vi "Network-Order Bytes To Words I64.vi"(1 "bytes in":u8[](array[numeric]) format="%02x") -> (0 "words out":i64[](array[numeric]) format="%x")   [LabVIEW 2020, in "NI_Bit Manipulation.lvlib"]
uses:
  <vilib>/Bit Manipulation/NI_Bit Manipulation.lvlib
  445b2e95-4c26-4098-854f-89dad29dbcf2.vi
  445b2e95-4c26-4098-854f-89dad29dbcf2.vi/567e058c-6714-4ee5-9ed8-7c8056630cc8.vi
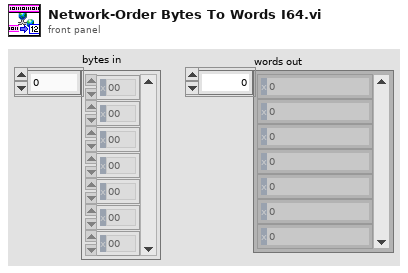
[diagram p1: front panel]
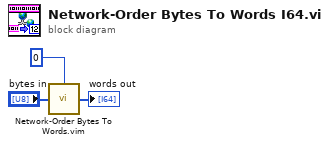
[diagram p0: block diagram]
diagram:
  n1 = call "Network-Order Bytes To Words.vim"("bytes in"="bytes in", "word type"=i64 0) -> ("words out"=→"words out":i64[])
